vi "Status FGV.vi"(7 "Live Status Ref":refnum<vi>, 8 "Error In":errorcluster, 9 "Status":string, 10 "Status FGV State":T1=enum."Set") -> (0 "Error Out":errorcluster, 2 "History":string, 3 "Log":string)   [LabVIEW 2020, in "LMH-LINX.lvlib"]
uses:
  LMH-LINX.lvlib
  Status FGV States.ctl
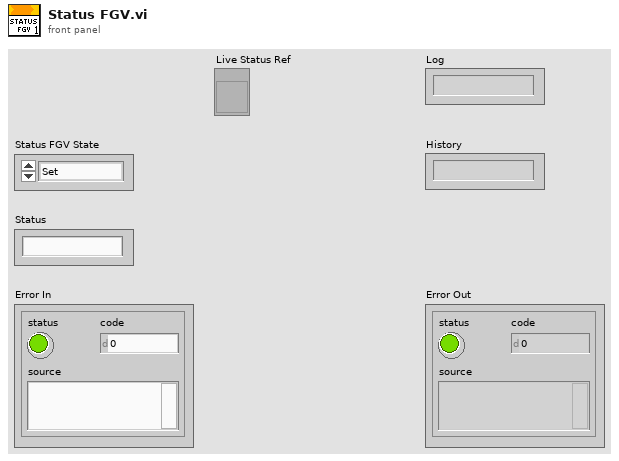
[diagram p1: front panel]
types:
  T1 = typedef "LMH-LINX.lvlib/Status FGV States.ctl" = enum16{"Init", "Append", "Append History Only", "Set", "Get"}
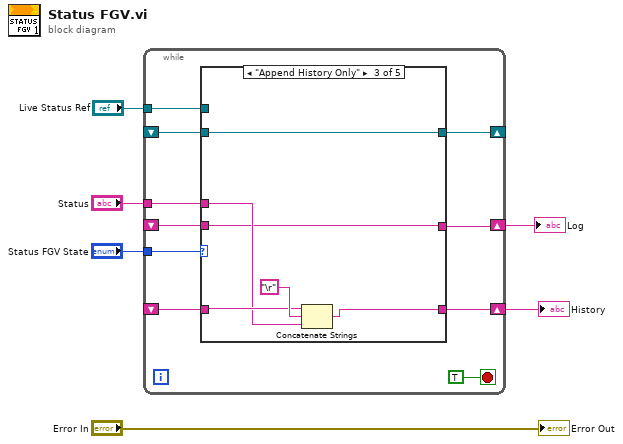
[diagram p0: block diagram]
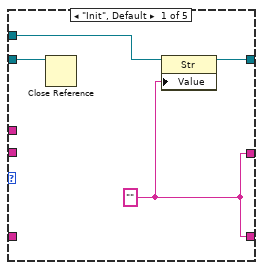
[diagram p2: hidden frame]
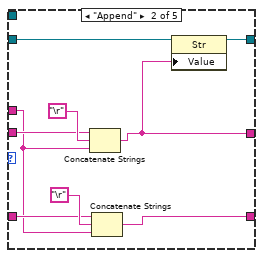
[diagram p3: hidden frame]
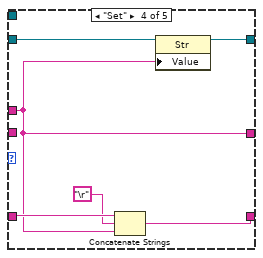
[diagram p4: hidden frame]
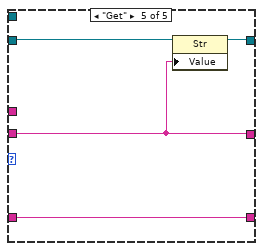
[diagram p5: hidden frame]
diagram:
  n1 = while {
    tunnel: "Status FGV State" -> [w16]
    shift-right: [w13] -> w4
    shift-left: _ -> [w15]
    tunnel: "Status" -> [w14]
    shift-right: [w11] -> w3
    shift-left: _ -> [w10]
    shift-right: [w7] -> _
    shift-left: _ -> [w9]
    tunnel: "Live Status Ref" -> [w8]
    stop <- TRUE stop-if-true
    n2 = case shown="\"Append History Only\"" w16 {
      tunnel: w15 -> [_ w26 w30 _ w42]
      tunnel: w14 -> [_ w24 w32 w36 _]
      tunnel: [w18 w21 w30 w36 w42] -> w13
      tunnel: [w18 w27 w31 w40 w45] -> w11
      tunnel: w10 -> [_ w25 w33 w41 w45]
      tunnel: w9 -> [w17 w23 w35 w37 w43]
      tunnel: w8 -> [w20 _ _ _ _]
      tunnel: [w19 w22 w35 w38 w44] -> w7
      frame "Init", Default {
        w18 = "" ("Status")
        n3 = Close Reference(reference=w17) -> ()  [unwired: 1 in, 1 out]
        n4 = property class="Str"(reference=w20, "Value"=w18) -> (reference out=w19:refnum<vi>)  [unwired: 1 in, 1 out]
      }
      frame "Append" {
        n5 = Concatenate Strings(w26, "\r", w24) -> (w21:string)
        n6 = Concatenate Strings(w25, "\r", w24) -> (w27:string)
        n7 = property class="Str"(reference=w23, "Value"=w21) -> (reference out=w22:refnum<vi>)  [unwired: 1 in, 1 out]
      }
      frame "Append History Only" {
        n8 = Concatenate Strings(w33, "\r", w32) -> (w31:string)
      }
      frame "Set" {
        n9 = Concatenate Strings(w41, "\r", w36) -> (w40:string)
        n10 = property class="Str"(reference=w37, "Value"=w36) -> (reference out=w38:refnum<vi>)  [unwired: 1 in, 1 out]
      }
      frame "Get" {
        n11 = property class="Str"(reference=w43, "Value"=w42) -> (reference out=w44:refnum<vi>)  [unwired: 1 in, 1 out]
      }
    }
  }
  "Log" <- w4
  "History" <- w3
  "Error Out" <- "Error In"
